vi "外观 2.vi"(0 "Data In":T6 caption="数据输入" format="%04x", 2 "Display State In":T4={"阀口名称"={"阀口名称自定义类型"=enum."自定义", "阀口自定义名称"={"V1"="V1", "V2"="V2", "V3"="V3", "V4"="V4", "V5"="V5", "V6"="V6", "V7"="V7", "V8"="V8", "V9"="V9", "V10"="V10", "V11"="V11", "V12"="V12", "V9-1"="V9-1", "V9-2"="V9-2", "COD慢速"="V9-2"}}} caption="显示状态输入", 3 "Container State":T5 caption="容器状态") -> (6 "Data Out":T6 caption="数据输出" format="%04x", 7 "Display State Out":T4={"阀口名称"={"阀口名称自定义类型"=enum."自定义", "阀口自定义名称"={"V1"="V1", "V2"="V2", "V3"="V3", "V4"="V4", "V5"="V5", "V6"="V6", "V7"="V7", "V8"="V8", "V9"="V9", "V10"="V10", "V11"="V11", "V12"="V12", "V9-1"="V9-1", "V9-2"="V9-2", "COD慢速"="V9-2"}}} caption="显示状态输出", 8 "Action":T3 caption="动作")   [LabVIEW 2016, in "调试控件V3.xctl"]
uses:
  <vilib>/_xctls/Container State.ctl
  <vilib>/_xctls/Action.ctl
  <vilib>/_xctls/XControlSupport.lvlib
panel:
  in  "项目输入":u16(ring) items=["总磷", "总氮", "氨氮", "磷酸盐", "硝氮", "亚硝氮", "硅酸盐", "硫化物", "COD"]
  in  "氨氮控温":bool
  in  "电磁阀2":bool
  in  "电磁阀1":bool
  in  "蠕动泵":bool
  in  "控温":enum32{"未选择", "消解", "恒温", "降温"}(radio)
  out "选项卡控件":enum32{"选项卡 1", "选项卡 2"}(tab)
  in  "COD慢速":bool
  in  "阀口选择":T1(radio)
  in  "V9-1":bool
  in  "V9-2":bool
  in  "灯":enum32{"未选择", "365", "520", "660", "氙灯/紫灯"}(radio)
  in  "ADC值":T2(radio)
  in  "注射泵":enum32{"等待", "复位", "注入", "注出"}(radio)=enum."注入"
  in  "数值":i16=4000
  # "外设"
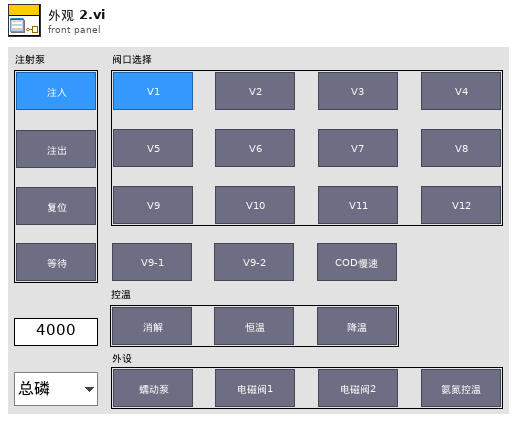
[diagram p1: front panel]
types:
  T1 = enum32{"V1", "V2", "V3", "V4", "V5", "V6", "V7", "V8", "V9", "V10", "V11", "V12"}
  T2 = enum32{"未选择", "ADC365", "ADC520", "ADC660", "光谱仪"}
  T3 = typedef "XControlSupport.lvlib/Action.ctl" = cluster{"Data Changed?":bool, "State Changed?":bool, "Action Name":string}
  T4 = typedef "调试控件V3.xctl/状态 2.ctl" = cluster{"阀口名称":cluster{"阀口名称自定义类型":enum16{"自定义", "微站总磷总氮", "微站总磷氨氮", "微站氨氮", "固定站总磷", "固定站总氮", "固定站氨氮", "原位总磷总氮", "原位总磷氨氮", "原位总磷", "原位总氮", "原位氨氮", "原位3N1P"}, "阀口自定义名称":cluster{"V1":string, "V2":string, "V3":string, "V4":string, "V5":string, "V6":string, "V7":string, "V8":string, "V9":string, "V10":string, "V11":string, "V12":string, "V9-1":string, "V9-2":string, "COD慢速":string}}}
  T5 = typedef "XControlSupport.lvlib/Container State.ctl" = cluster{"Indicator?":bool, "Run Mode?":bool, " Refnum":refnum<vi>}
  T6 = typedef "调试控件V3.xctl/数据 2.ctl" = u16[]
  T7 = cluster{"默认名称":cluster{"V1":string, "V2":string, "V3":string, "V4":string, "V5":string, "V6":string, "V7":string, "V8":string, "V9":string, "V10":string, "V11":string, "V12":string, "V9-1":string, "V9-2":string, "COD慢速":string}, "微站总磷总氮":cluster{"V1":string, "V2":string, "V3":string, "V4":string, "V5":string, "V6":string, "V7":string, "V8":string, "V9":string, "V10":string, "V11":string, "V12":string, "V9-1":string, "V9-2":string, "COD慢速":string}, "微站总磷氨氮":cluster{"V1":string, "V2":string, "V3":string, "V4":string, "V5":string, "V6":string, "V7":string, "V8":string, "V9":string, "V10":string, "V11":string, "V12":string, "V9-1":string, "V9-2":string, "COD慢速":string}, "微站氨氮":cluster{"V1":string, "V2":string, "V3":string, "V4":string, "V5":string, "V6":string, "V7":string, "V8":string, "V9":string, "V10":string, "V11":string, "V12":string, "V9-1":string, "V9-2":string, "COD慢速":string}, "固定站总磷":cluster{"V1":string, "V2":string, "V3":string, "V4":string, "V5":string, "V6":string, "V7":string, "V8":string, "V9":string, "V10":string, "V11":string, "V12":string, "V9-1":string, "V9-2":string, "COD慢速":string}, "固定站总氮":cluster{"V1":string, "V2":string, "V3":string, "V4":string, "V5":string, "V6":string, "V7":string, "V8":string, "V9":string, "V10":string, "V11":string, "V12":string, "V9-1":string, "V9-2":string, "COD慢速":string}, "固定站氨氮":cluster{"V1":string, "V2":string, "V3":string, "V4":string, "V5":string, "V6":string, "V7":string, "V8":string, "V9":string, "V10":string, "V11":string, "V12":string, "V9-1":string, "V9-2":string, "COD慢速":string}, "原位总磷总氮":cluster{"V1":string, "V2":string, "V3":string, "V4":string, "V5":string, "V6":string, "V7":string, "V8":string, "V9":string, "V10":string, "V11":string, "V12":string, "V9-1":string, "V9-2":string, "COD慢速":string}, "原位总磷氨氮":cluster{"V1":string, "V2":string, "V3":string, "V4":string, "V5":string, "V6":string, "V7":string, "V8":string, "V9":string, "V10":string, "V11":string, "V12":string, "V9-1":string, "V9-2":string, "COD慢速":string}, "原位总磷":cluster{"V1":string, "V2":string, "V3":string, "V4":string, "V5":string, "V6":string, "V7":string, "V8":string, "V9":string, "V10":string, "V11":string, "V12":string, "V9-1":string, "V9-2":string, "COD慢速":string}, "原位总氮":cluster{"V1":string, "V2":string, "V3":string, "V4":string, "V5":string, "V6":string, "V7":string, "V8":string, "V9":string, "V10":string, "V11":string, "V12":string, "V9-1":string, "V9-2":string, "COD慢速":string}, "原位氨氮":cluster{"V1":string, "V2":string, "V3":string, "V4":string, "V5":string, "V6":string, "V7":string, "V8":string, "V9":string, "V10":string, "V11":string, "V12":string, "V9-1":string, "V9-2":string, "COD慢速":string}, "原位3N1P":cluster{"V1":string, "V2":string, "V3":string, "V4":string, "V5":string, "V6":string, "V7":string, "V8":string, "V9":string, "V10":string, "V11":string, "V12":string, "V9-1":string, "V9-2":string, "COD慢速":string}}
  T8 = enum16{"自定义", "微站总磷总氮", "微站总磷氨氮", "微站氨氮", "固定站总磷", "固定站总氮", "固定站氨氮", "原位总磷总氮", "原位总磷氨氮", "原位总磷", "原位总氮", "原位氨氮", "原位3N1P"}
  T9 = cluster{"V1":string, "V2":string, "V3":string, "V4":string, "V5":string, "V6":string, "V7":string, "V8":string, "V9":string, "V10":string, "V11":string, "V12":string, "V9-1":string, "V9-2":string, "COD慢速":string}
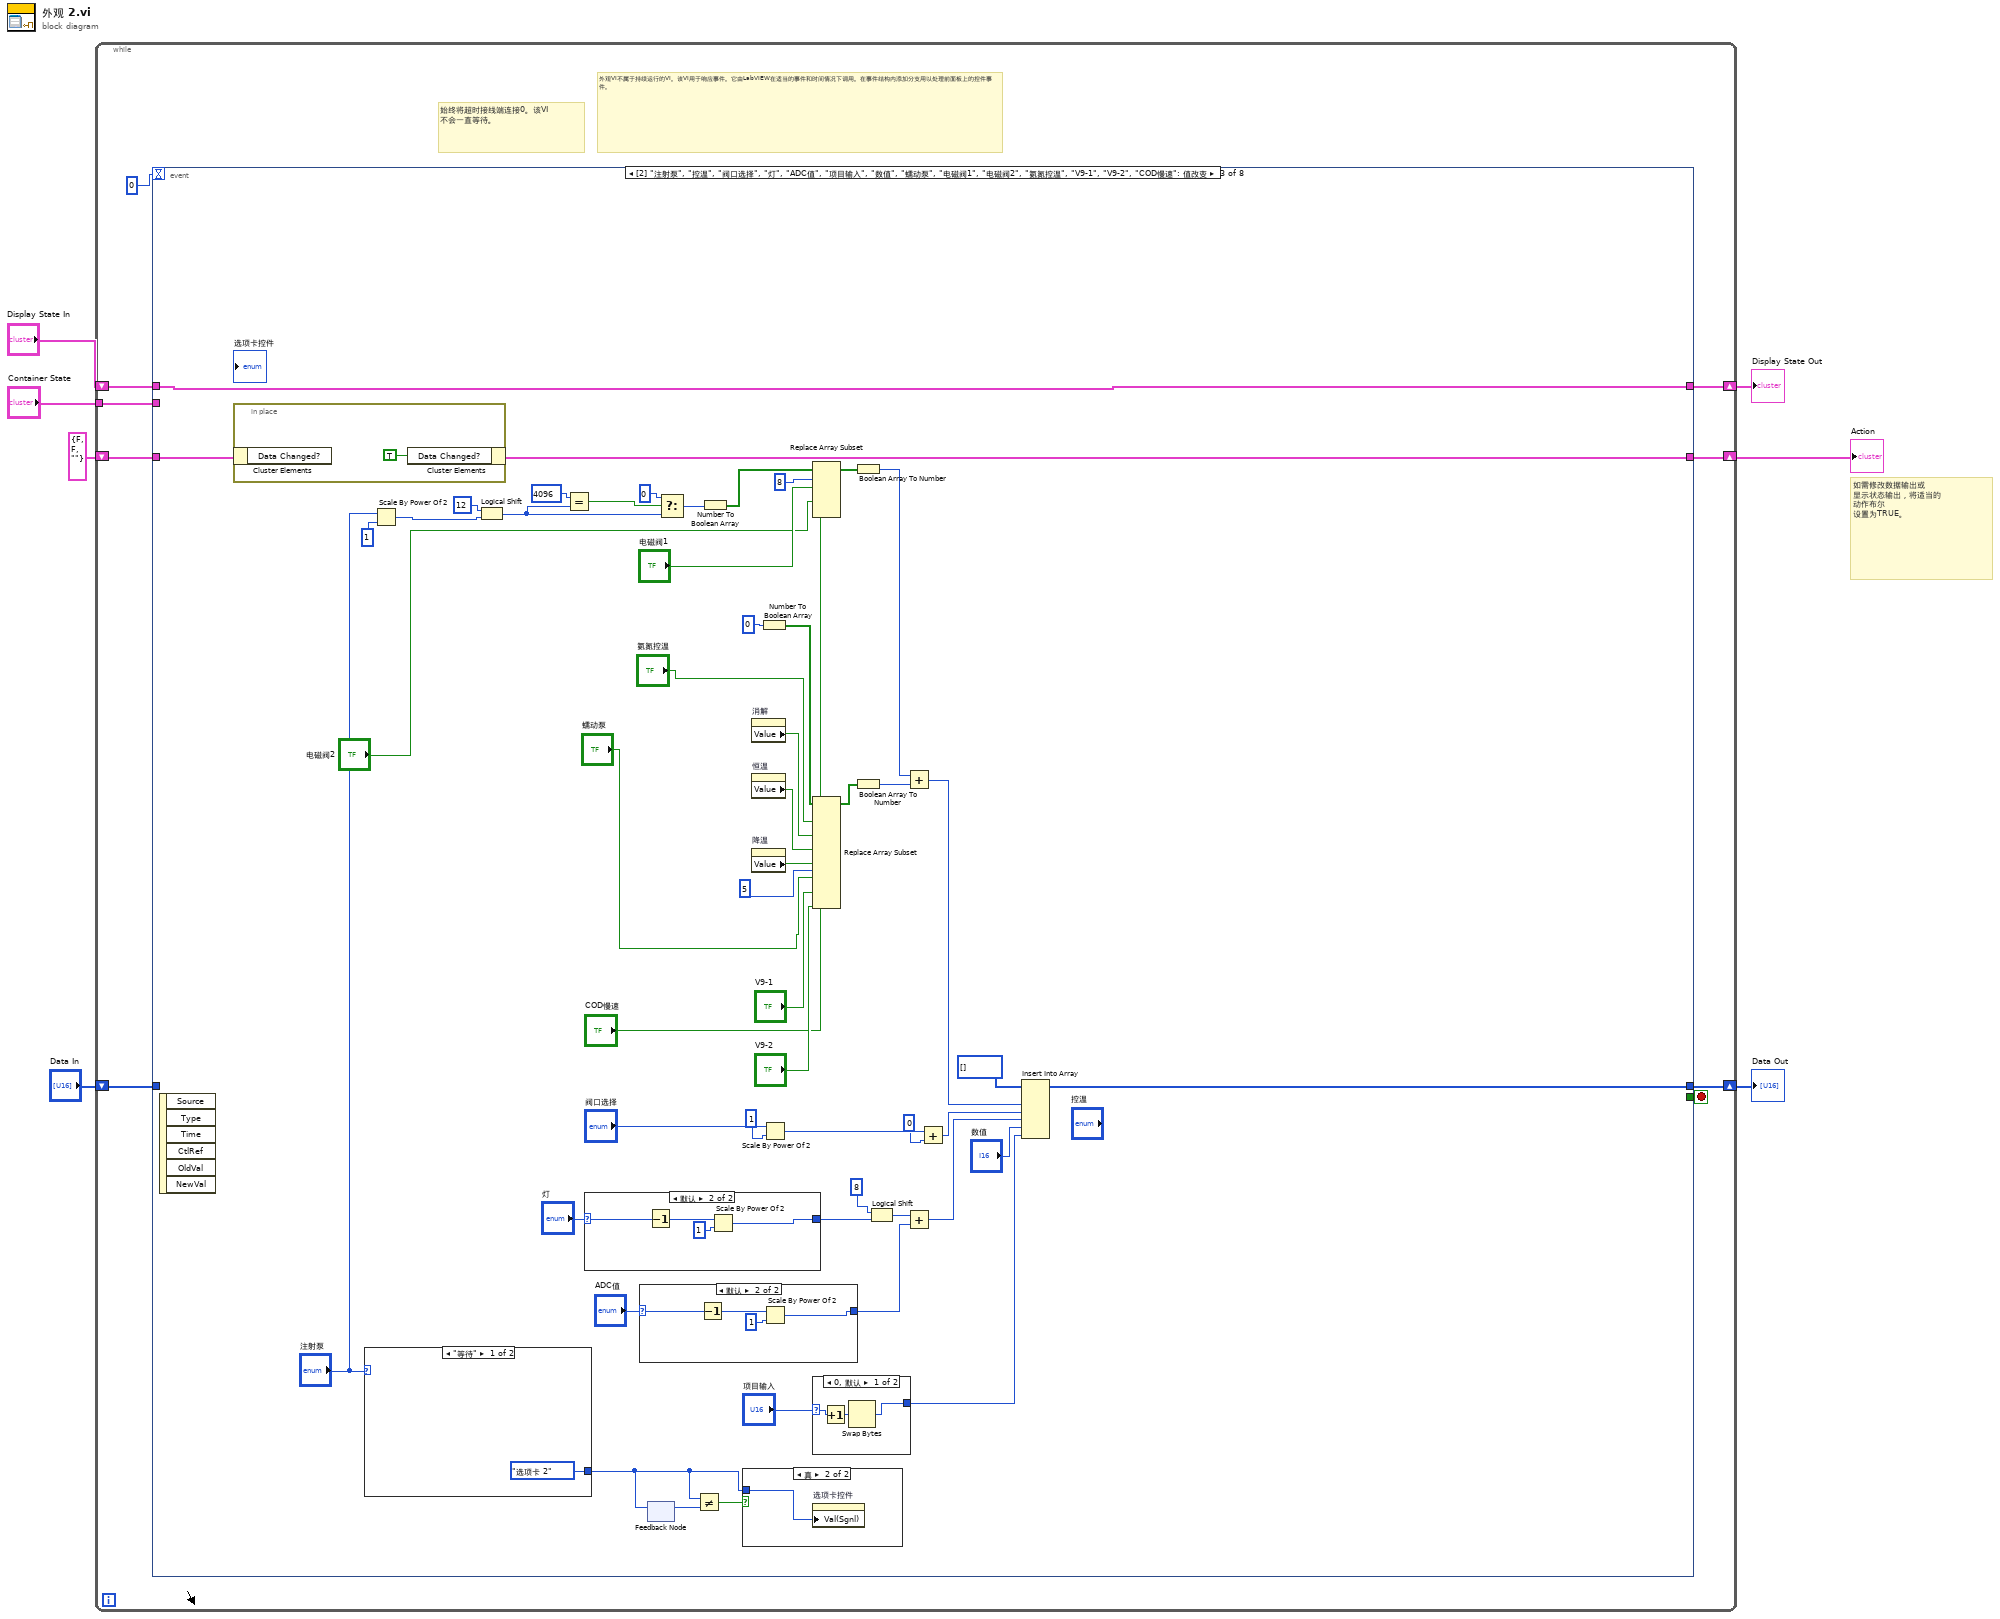
[diagram p0: block diagram]
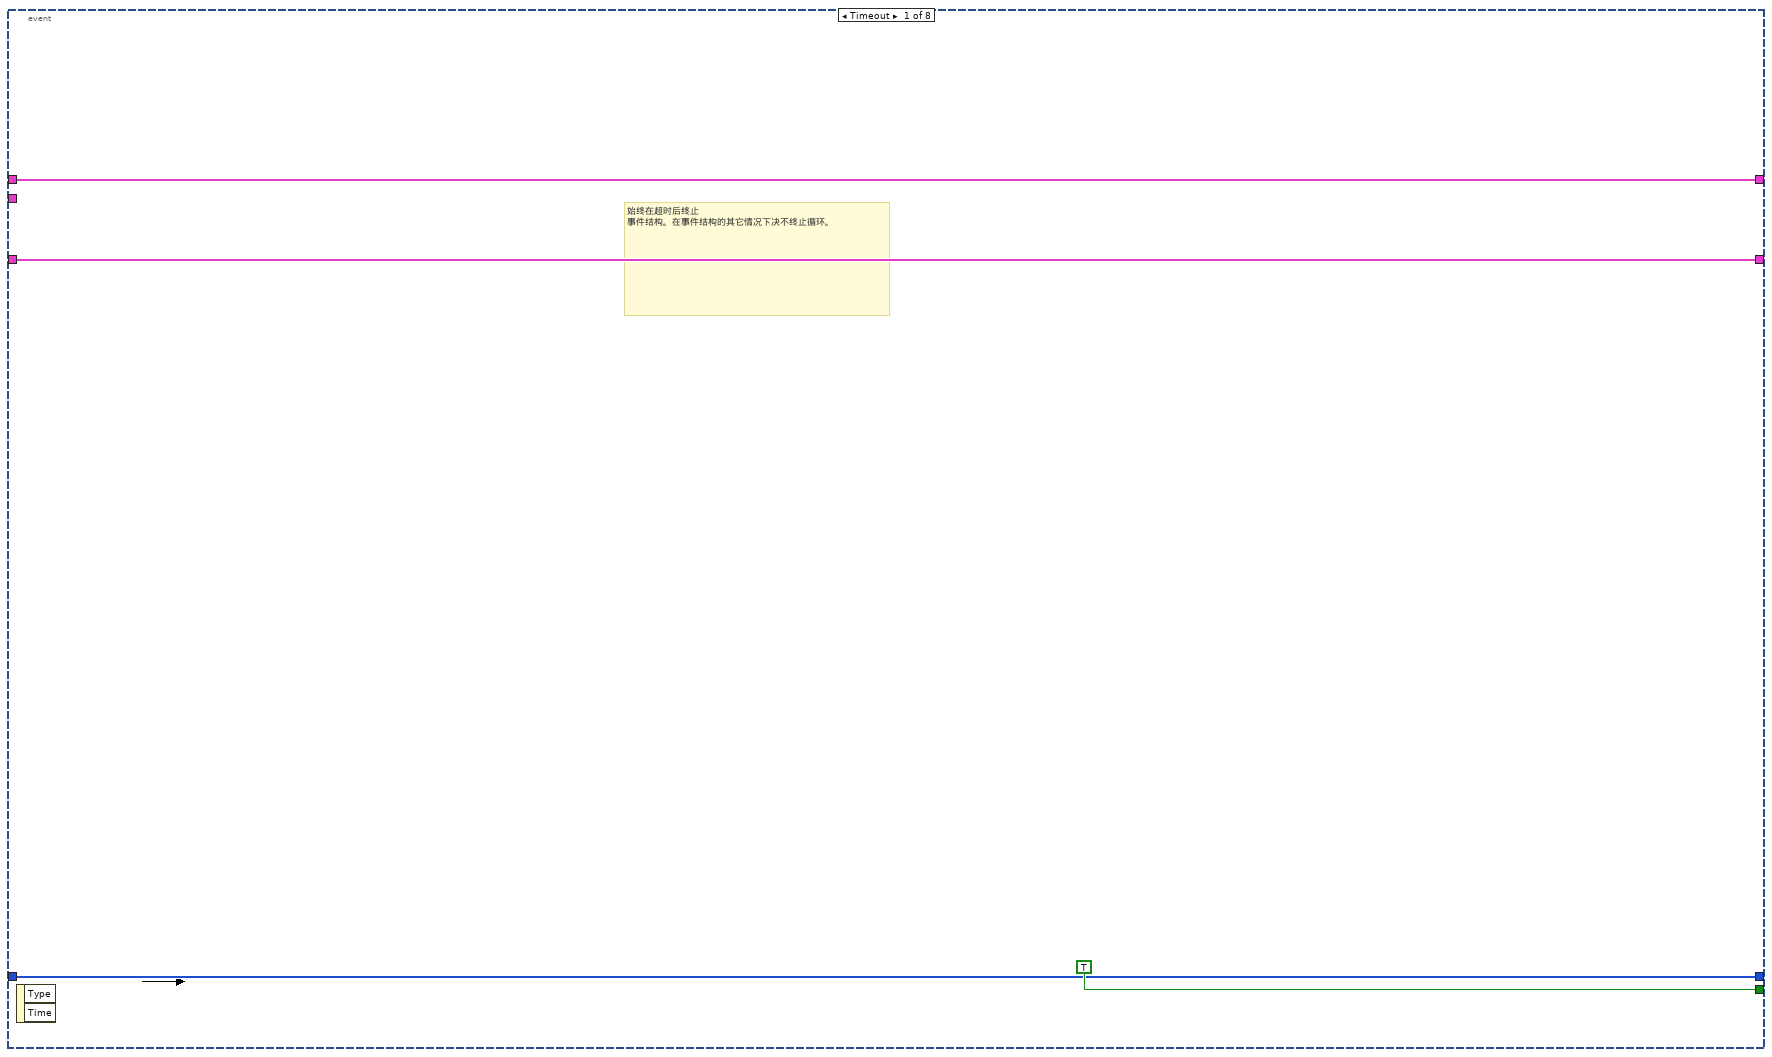
[diagram p2: hidden frame]
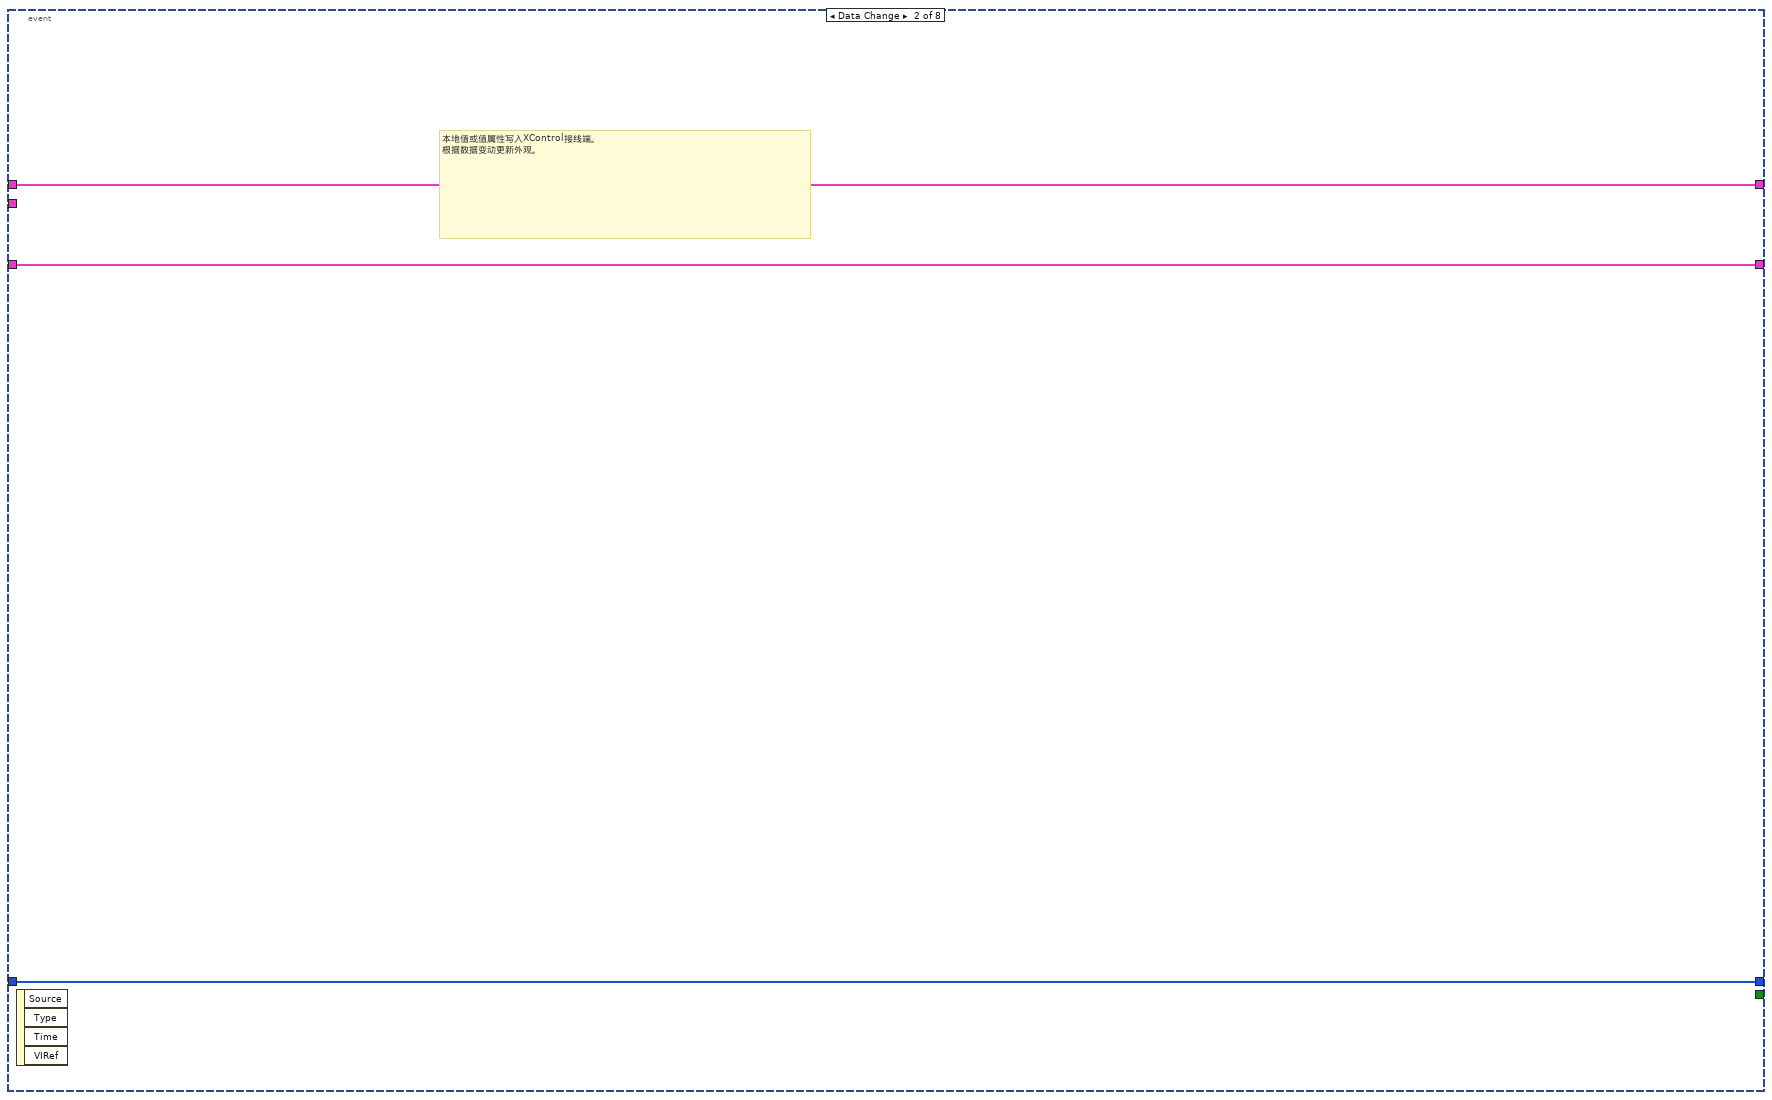
[diagram p3: hidden frame]
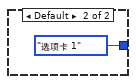
[diagram p5: hidden frame]
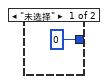
[diagram p6: hidden frame]
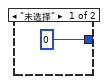
[diagram p7: hidden frame]
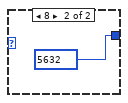
[diagram p8: hidden frame]
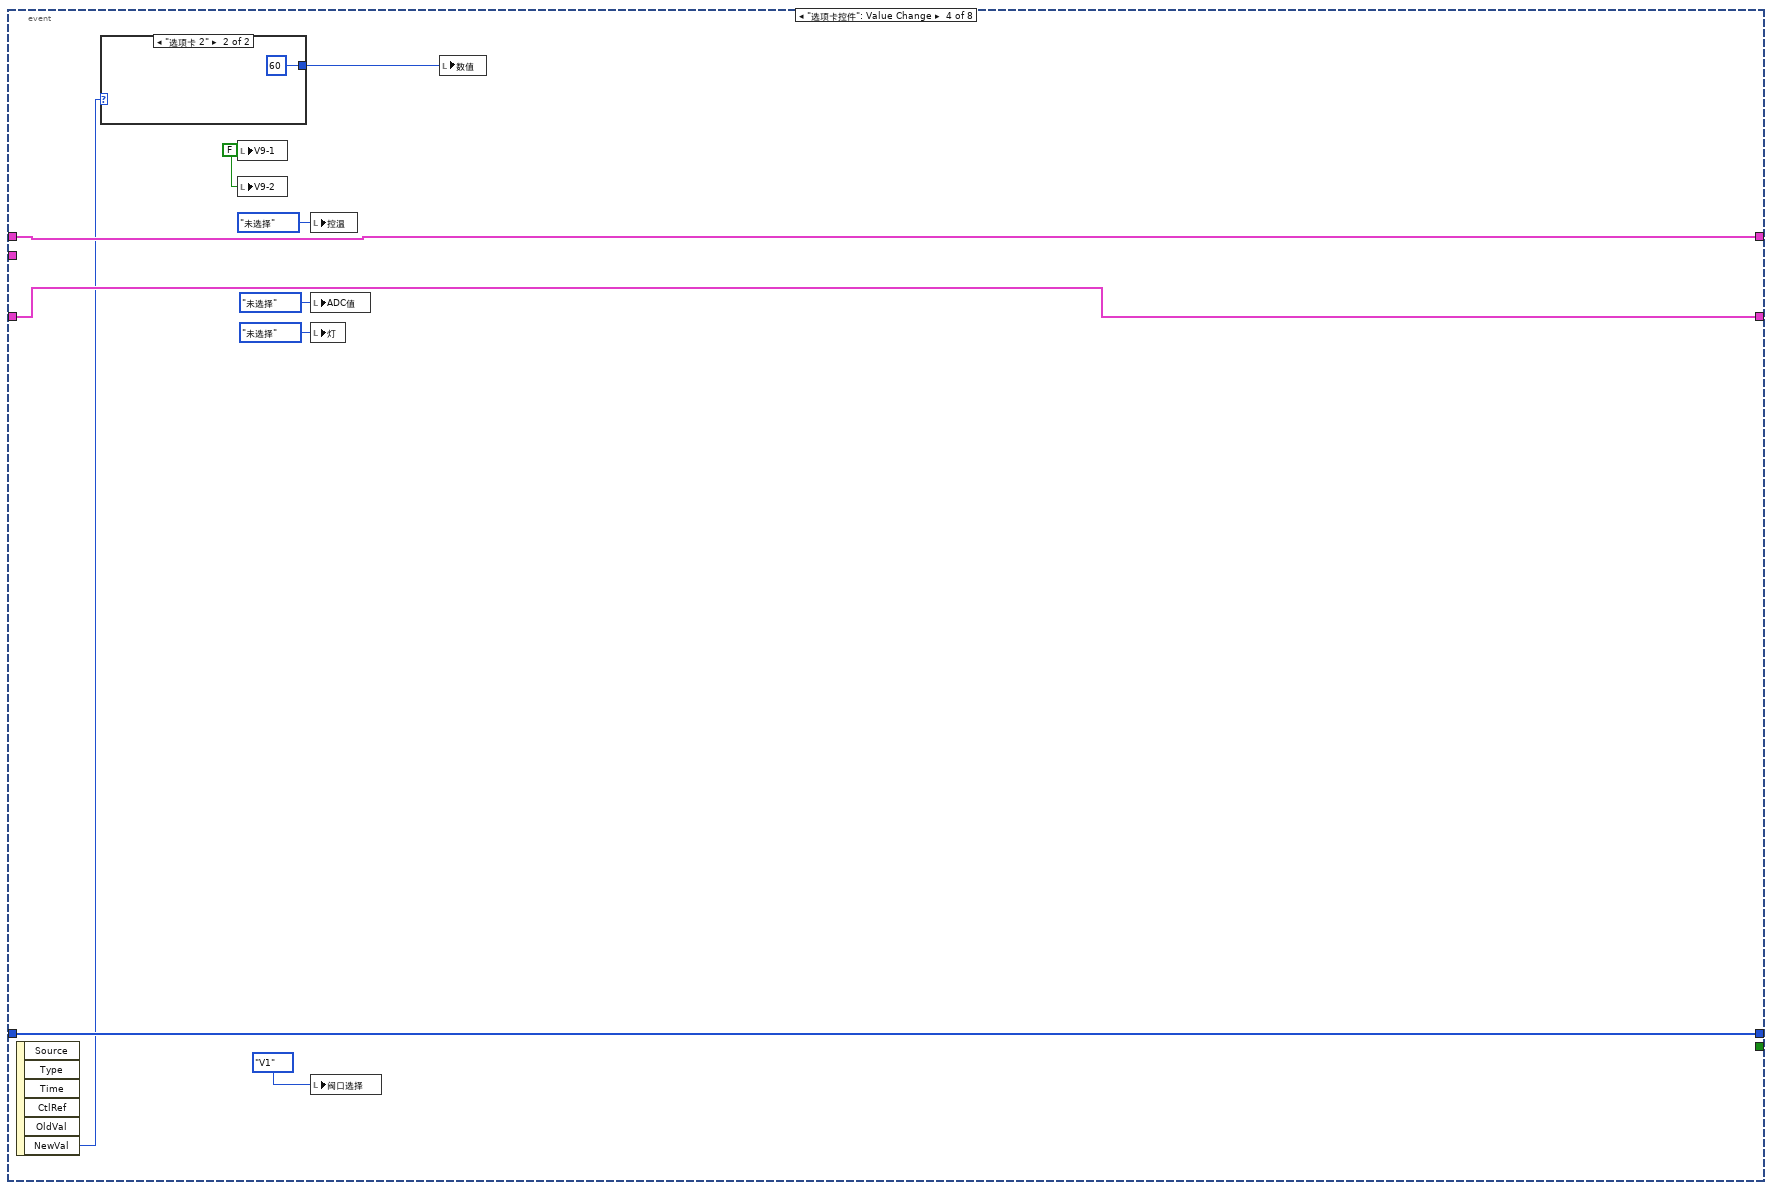
[diagram p9: hidden frame]
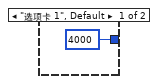
[diagram p10: hidden frame]
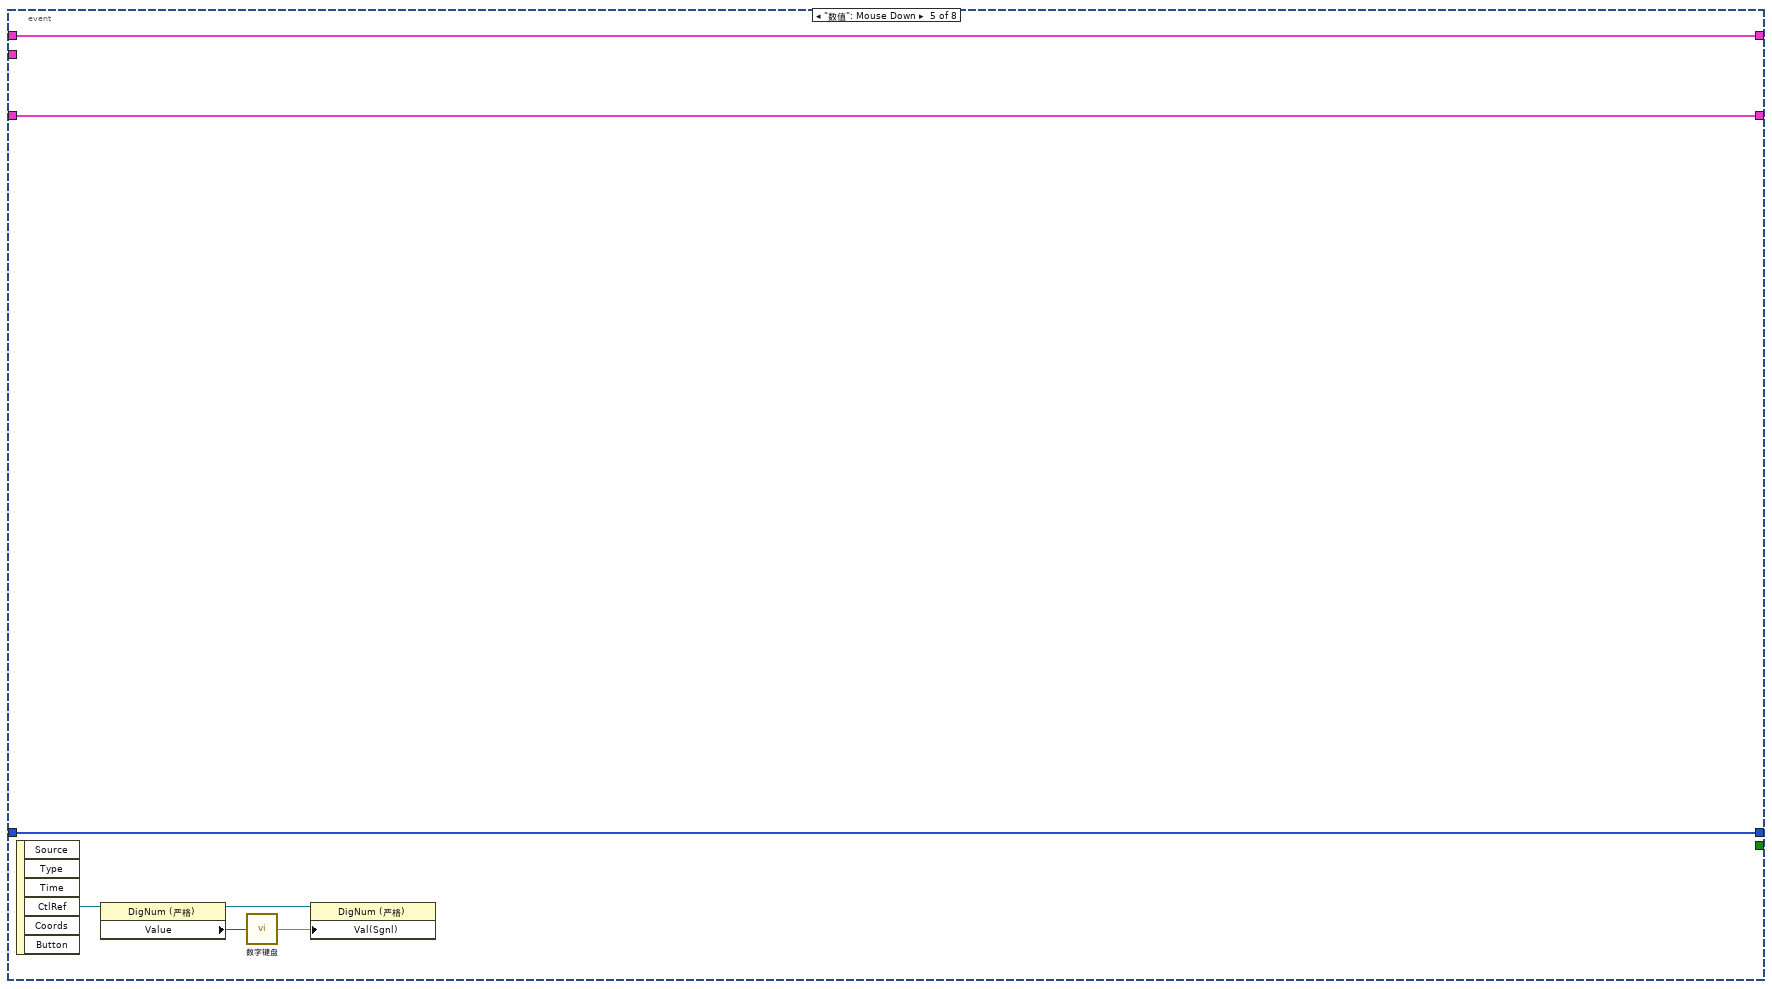
[diagram p11: hidden frame]
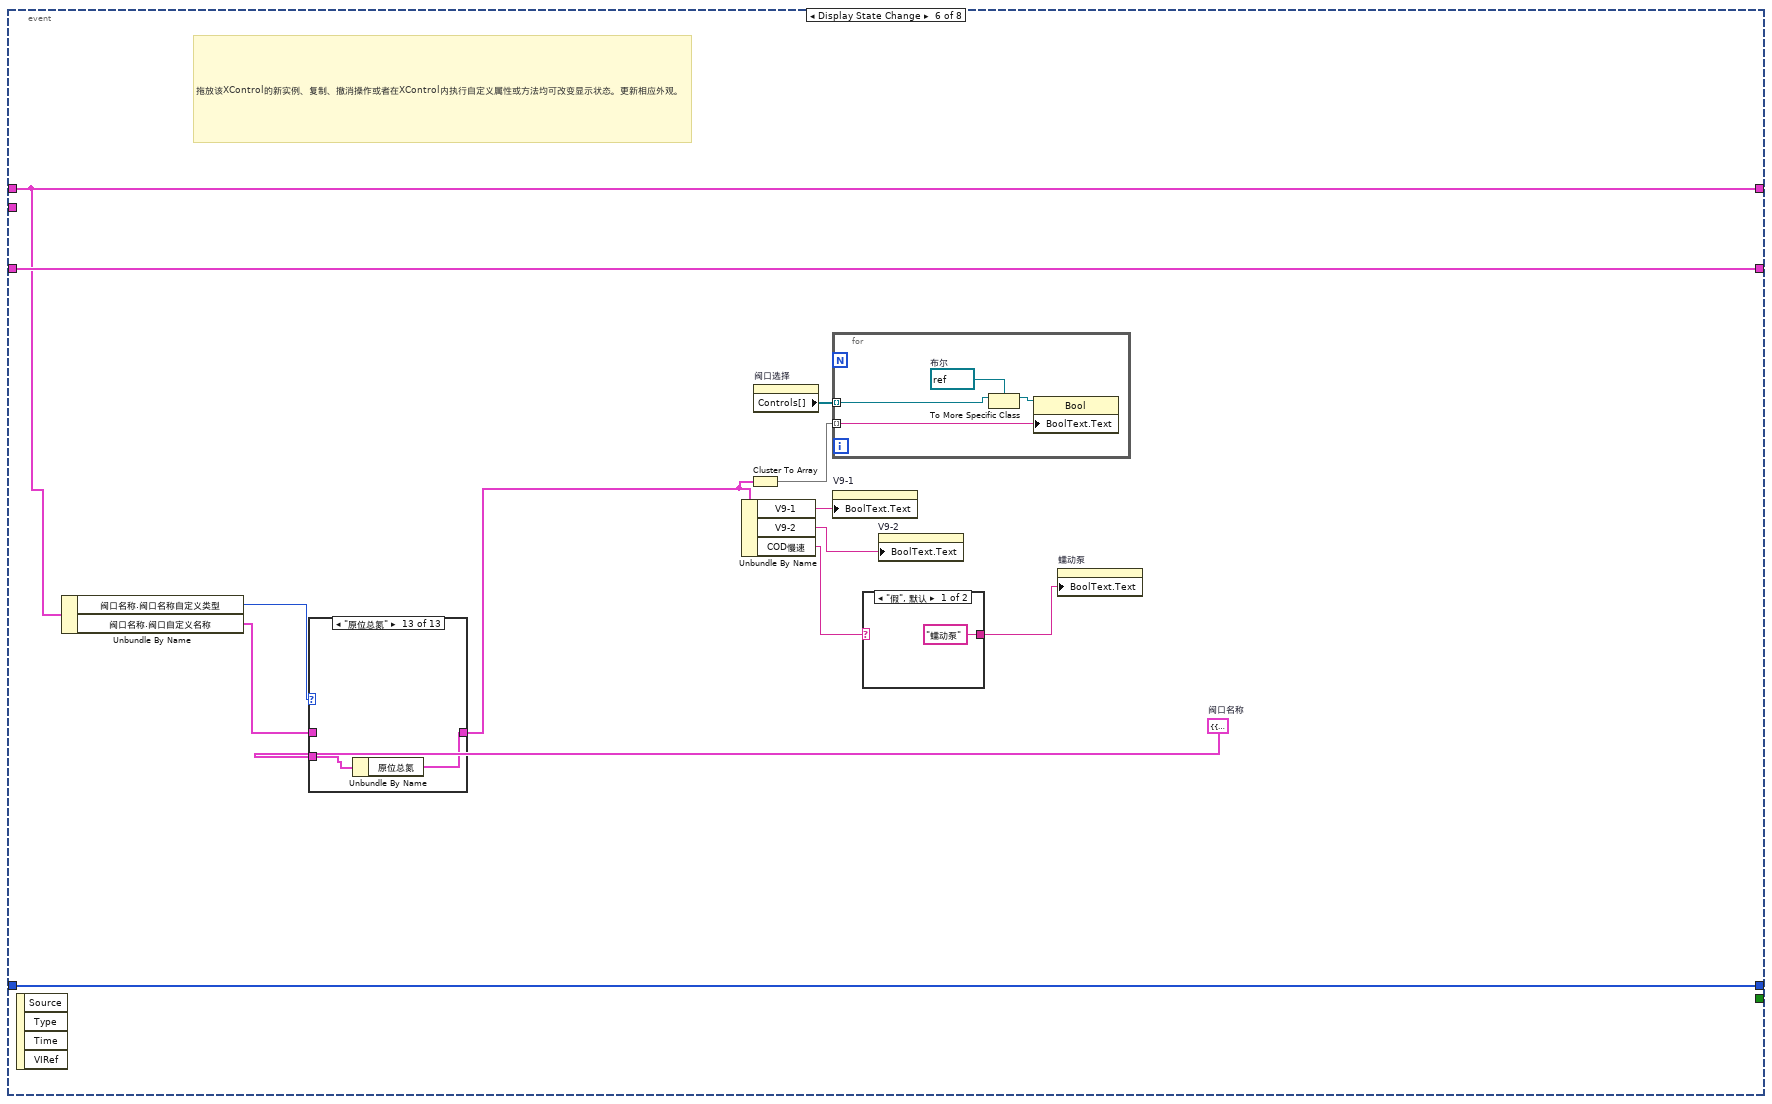
[diagram p12: hidden frame]
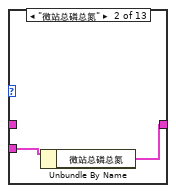
[diagram p15: hidden frame]
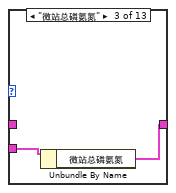
[diagram p16: hidden frame]
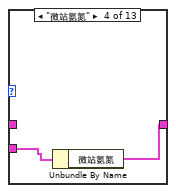
[diagram p17: hidden frame]
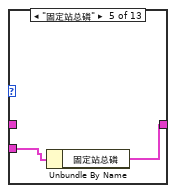
[diagram p18: hidden frame]
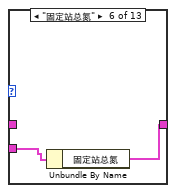
[diagram p19: hidden frame]
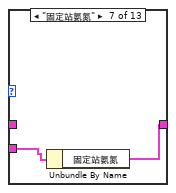
[diagram p20: hidden frame]
diagram:
  # "如需修改数据输出或\n显示状态输出，将适当的\n动作布尔\n设置为TRUE。"
  n1 = while {
    shift-right: [w15] -> w4
    shift-left: "Display State In" -> [w16]
    tunnel: "Container State" -> [w12]
    shift-right: [w10] -> w7
    shift-left: "Data In" -> [w11]
    shift-right: [w8] -> w2
    shift-left: T3 {"Data Changed?"=FALSE, "State Changed?"=FALSE, "Action Name"=""} ("Action") -> [w9]
    stop <- w14 stop-if-true
    # "外观VI不属于持续运行的VI。该VI用于响应事件。它由LabVIEW在适当的事件和时间情况下调用。在事件结构内添加分支用以处理前面板上的控件事件。"
    # "始终将超时接线端连接0。该VI\n不会一直等待。"
    n2 = event shown="[2] \"注射泵\", \"控温\", \"阀口选择\", \"灯\", \"ADC值\", \"项目输入\", \"数值\", \"蠕动泵\", \"电磁阀1\", \"电磁阀2\", \"氨氮控温\", \"V9-1\", \"V9-2\", \"COD慢速\": 值改变" {
      selector: _ -> [_ _ _ _ _ _ _ _]
      dyn-events: _ -> [_ _ _ _ _ _ _ _]
      timeout: 0 -> [_ _ _ _ _ _ _ _]
      tunnel: w16 -> [w18 w22 w75 w103 w112 w119 w159 w163]
      tunnel: [w18 w22 w75 w103 w112 w119 w159 w163] -> w15
      tunnel: [TRUE _ _ _ _ _ _ _] -> w14
      tunnel: w12 -> [_ _ _ _ _ _ w160 w164]
      tunnel: w11 -> [w17 w23 _ w102 w111 w125 w158 w162]
      tunnel: [w17 w23 w51 w102 w111 w125 w158 w162] -> w10
      tunnel: [w19 w21 w73 w101 w110 w124 w157 w161] -> w8
      tunnel: w9 -> [w19 w21 w74 w101 w110 w124 w157 w161]
      event Timeout {
        # "始终在超时后终止\n事件结构。在事件结构的其它情况下决不终止循环。"
        n3 = event-data() -> ()  [unwired: 1 in, 2 out]
      }
      event Data Change {
        # "本地值或值属性写入XControl接线端。\n根据数据变动更新外观。"
        n4 = event-data() -> ()  [unwired: 1 in, 4 out]
      }
      event "注射泵", "控温", "阀口选择", "灯", "ADC值", "项目输入", "数值", "蠕动泵", "电磁阀1", "电磁阀2", "氨氮控温", "V9-1", "V9-2", "COD慢速": Value Change {
        n5 = event-data() -> ()  [unwired: 1 in, 6 out]
        n6 = in-place {
          n7 = in-place-cluster #1(w74) -> ()  [unwired: 1 out]
          n8 = in-place-cluster #1("Data Changed?"=TRUE) -> (w73:T3)
        }
        n9 = case shown="\"等待\"" "注射泵" {
          tunnel: [enum32{"选项卡 1", "选项卡 2"}."选项卡 2" ("选项卡控件") enum32{"选项卡 1", "选项卡 2"}."选项卡 1" ("选项卡控件")] -> w45
          frame "等待" {
          }
          frame Default {
          }
        }
        n10 = Scale By Power Of 2(n="注射泵", x=i16 1 ("y")) -> (x*2^n=w59:i16)
        n11 = Logical Shift(y=i16 12, x=w59) -> (x << y=w64:i16)
        n12 = Equal?(x=u32 4096 ("t"), y=w64) -> (x = y?=w72:bool)
        n13 = case shown="默认" "灯" {
          selector: "灯" -> [_ w86]
          tunnel: [i16 0 ("y") w88] -> w56
          frame "未选择" {
          }
          frame Default {
            n14 = Decrement(x=w86) -> (x-1=w87:enum32{"未选择", "365", "520", "660", "氙灯/紫灯"})
            n15 = Scale By Power Of 2(n=w87, x=i16 1 ("y")) -> (x*2^n=w88:i16)
          }
        }
        n16 = case shown="默认" "ADC值" {
          selector: "ADC值" -> [_ w81]
          tunnel: [i16 0 ("y") w83] -> w55
          frame "未选择" {
          }
          frame Default {
            n17 = Decrement(x=w81) -> (x-1=w82:T2)
            n18 = Scale By Power Of 2(n=w82, x=i16 1 ("y")) -> (x*2^n=w83:i16)
          }
        }
        n19 = feedback-in #2(w45) -> ()
        n20 = feedback #2() -> (w47:enum32{"选项卡 1", "选项卡 2"})  [unwired: 1 in]
        n21 = Select(t=u32 0, s=w72, f=w64) -> (s? t:f=w41:u32)
        n22 = Not Equal?(x=w45, y=w47) -> (x != y?=w46:bool)
        n23 = Number To Boolean Array(number=w41) -> (Boolean array=w40:bool[])
        n24 = case shown="真" w46 {
          tunnel: w45 -> [_ w76]
          frame False {
          }
          frame True {
            n25 = property on="选项卡控件" class="TabCtl (严格)"("Val(Sgnl)"=w76) -> ()  [unwired: 2 in, 2 out]
          }
        }
        n26 = property on="消解" class="Bool (严格)"() -> ("Value"=w36:bool)  [unwired: 2 in, 2 out]
        n27 = property on="恒温" class="Bool (严格)"() -> ("Value"=w35:bool)  [unwired: 2 in, 2 out]
        n28 = property on="降温" class="Bool (严格)"() -> ("Value"=w34:bool)  [unwired: 2 in, 2 out]
        n29 = Number To Boolean Array(number=u16 0) -> (Boolean array=w31:bool[])
        n30 = Scale By Power Of 2(n="阀口选择", x=i16 1 ("y")) -> (x*2^n=w58:i16)
        n31 = Replace Array Subset(array=w40, new element #1="电磁阀1", index #1=8 ("索引"), new element #2="电磁阀2", new element #3="COD慢速") -> (w39:bool[])  [unwired: 2 in]
        n32 = Replace Array Subset(array=w31, new element #1="氨氮控温", new element #2=w36, new element #3=w35, new element #4=w34, new element #5="蠕动泵", index #5=5 ("索引"), new element #6="V9-1", new element #7="V9-2") -> (w48:bool[])  [unwired: 6 in]
        n33 = case shown="0, 默认" "项目输入" {
          selector: "项目输入" -> [w91 _]
          tunnel: [w90 5632] -> w61
          frame 0, Default {
            n34 = Increment(x=w91) -> (x+1=w89:u16)
            n35 = Swap Bytes(anything=w89) -> (byte swapped=w90:u16)
          }
          frame 8 {
          }
        }
        n36 = Boolean Array To Number(Boolean array=w39) -> (number=w38:u32)
        n37 = Boolean Array To Number(Boolean array=w48) -> (number=w44:u32)
        n38 = Logical Shift(y=i16 8, x=w56) -> (x << y=w70:i16)
        n39 = Add(x=w38, y=w44) -> (x+y=w67:u32)
        n40 = Add(x=w70, y=w55) -> (x+y=w66:i16)
        n41 = Add(x=w58, y=i16 0) -> (x+y=w57:i16)
        n42 = Insert Into Array(array=u16[] [] ("数组"), new element #1=w67, new element #2=w57, new element #3=w66, new element #4="数值", new element #5=w61) -> (w51:u16[])  [unwired: 1 in]
      }
      event "选项卡控件": Value Change {
        w97 = FALSE ("V9-1")
        n43 = event-data() -> ("NewVal"=w100:enum32{"选项卡 1", "选项卡 2"})  [unwired: 1 in, 5 out]
        n44 = case shown="\"选项卡 2\"" w100 {
          tunnel: [i16 4000 ("数值") i16 60 ("数值")] -> w99
          frame "选项卡 1", Default {
          }
          frame "选项卡 2" {
          }
        }
        n45 = local write "V9-1"(w97) -> ()
        n46 = local write "V9-2"(w97) -> ()
        n47 = local write "控温"(enum32{"未选择", "消解", "恒温", "降温"}."未选择" ("控温")) -> ()
        n48 = local write "ADC值"(T2."未选择" ("ADC值")) -> ()
        n49 = local write "灯"(enum32{"未选择", "365", "520", "660", "氙灯/紫灯"}."未选择" ("灯")) -> ()
        n50 = local write "阀口选择"(T1."V1" ("阀口选择")) -> ()
        n51 = local write "数值"(w99) -> ()
      }
      event "数值": Mouse Down {
        n52 = event-data() -> ("CtlRef"=w109:refnum<vi>)  [unwired: 1 in, 5 out]
        n53 = property class="DigNum (严格)"(reference=w109) -> (reference out=w108:refnum<vi>, "Value"=w107:i16)  [unwired: 1 in, 1 out]
        n54 = call "数字键盘.vi"("OldNumber"=w107) -> ("NewNumber"=w106:sgl)
        n55 = property class="DigNum (严格)"(reference=w108, "Val(Sgnl)"=w106) -> ()  [unwired: 1 in, 2 out]
      }
      event Display State Change {
        w116 = T7 {"默认名称"={"V1"="V1", "V2"="V2", "V3"="V3", "V4"="V4", "V5"="V5", "V6"="V6", "V7"="V7", "V8"="V8", "V9"="V9", "V10"="V10", "V11"="V11", "V12"="V12", "V9-1"="V9-1", "V9-2"="V9-2", "COD慢速"="COD慢速"}, "微站总磷总氮"={"V1"="TA", "V2"="TB", "V3"="TC", "V4"="PA", "V5"="PB", "V6"="零点核查", "V7"="跨度核查", "V8"="纯水", "V9"="水样", "V10"="消解", "V11"="总氮比色", "V12"="总磷比色/废液", "V9-1"="加标回收", "V9-2"="标样核查", "COD慢速"="COD慢速"}, "微站总磷氨氮"={"V1"="NA", "V2"="NB", "V3"="NC", "V4"="TB", "V5"="PA", "V6"="PB", "V7"="跨度核查", "V8"="纯水", "V9"="水样", "V10"="消解", "V11"="空气", "V12"="比色/废液", "V9-1"="加标回收", "V9-2"="标样核查", "COD慢速"="COD慢速"}, "微站氨氮"={"V1"="NA", "V2"="NB", "V3"="NC", "V4"="零点核查", "V5"="跨度核查", "V6"="空气", "V7"="纯水", "V8"="水样", "V9"="排液", "V10"="V10", "V11"="V11", "V12"="V12", "V9-1"="加标回收", "V9-2"="标样核查", "COD慢速"="COD慢速"}, "固定站总磷"={"V1"="TB", "V2"="PA", "V3"="PB", "V4"="排液", "V5"="标样核查", "V6"="零点核查", "V7"="跨度核查", "V8"="纯水", "V9"="水样/加标", "V10"="消解", "V11"="空气", "V12"="总磷比色/废液", "V9-1"="V9-1", "V9-2"="V9-2", "COD慢速"="COD慢速"}, "固定站总氮"={"V1"="TA", "V2"="TB", "V3"="TC", "V4"="排液", "V5"="标样核查", "V6"="零点核查", "V7"="跨度核查", "V8"="纯水", "V9"="水样/加标", "V10"="消解", "V11"="总氮比色", "V12"="废液", "V9-1"="V9-1", "V9-2"="V9-2", "COD慢速"="COD慢速"}, "固定站氨氮"={"V1"="NA", "V2"="NB", "V3"="NC", "V4"="零点核查", "V5"="跨度核查", "V6"="空气", "V7"="纯水", "V8"="水样", "V9"="排液", "V10"="V10", "V11"="V11", "V12"="V12", "V9-1"="加标回收", "V9-2"="标样核查", "COD慢速"="COD慢速"}, "原位总磷总氮"={"V1"="TA", "V2"="TB", "V3"="TC", "V4"="PA", "V5"="PB", "V6"="零点核查", "V7"="跨度核查", "V8"="纯水", "V9"="水样", "V10"="消解", "V11"="总氮比色", "V12"="总磷比色/废液", "V9-1"="V9-1", "V9-2"="V9-2", "COD慢速"="COD慢速"}, "原位总磷氨氮"={"V1"="NA", "V2"="NB", "V3"="NC", "V4"="TB", "V5"="PA", "V6"="PB", "V7"="跨度核查", "V8"="纯水", "V9"="水样", "V10"="消解", "V11"="空气", "V12"="比色/废液", "V9-1"="V9-1", "V9-2"="V9-2", "COD慢速"="COD慢速"}, "原位总磷"={"V1"="TB", "V2"="PA", "V3"="PB", "V4"="排液", "V5"="标样核查", "V6"="零点核查", "V7"="跨度核查", "V8"="纯水", "V9"="水样/加标", "V10"="消解", "V11"="空气", "V12"="总磷比色/废液", "V9-1"="V9-1", "V9-2"="V9-2", "COD慢速"="COD慢速"}, "原位总氮"={"V1"="TA", "V2"="TB", "V3"="TC", "V4"="排液", "V5"="标样核查", "V6"="零点核查", "V7"="跨度核查", "V8"="纯水", "V9"="水样/加标", "V10"="消解", "V11"="总氮比色", "V12"="废液", "V9-1"="V9-1", "V9-2"="V9-2", "COD慢速"="COD慢速"}, "原位氨氮"={"V1"="NA", "V2"="NB", "V3"="NC", "V4"="零点核查", "V5"="跨度核查", "V6"="空气", "V7"="纯水", "V8"="水样", "V9"="排液", "V10"="V10", "V11"="V11", "V12"="V12", "V9-1"="加标回收", "V9-2"="标样核查", "COD慢速"="COD慢速"}, "原位3N1P"={"V1"="NAB", "V2"="PA", "V3"="PB", "V4"="OA", "V5"="OB", "V6"="RA", "V7"="空气", "V8"="纯水", "V9"="水样", "V10"="紫外还原", "V11"="氨氮比色", "V12"="排液/比色", "V9-1"="V9-1", "V9-2"="V9-2", "COD慢速"="COD慢速"}}  # 阀口名称
        # "拖放该XControl的新实例、复制、撤消操作或者在XControl内执行自定义属性或方法均可改变显示状态。更新相应外观。"
        n56 = event-data() -> ()  [unwired: 1 in, 4 out]
        n57 = Unbundle By Name(w119) -> ("阀口名称.阀口名称自定义类型"=w118:T8, "阀口名称.阀口自定义名称"=w117:T9)
        n58 = case shown="\"原位总氮\"" w118 {
          tunnel: w117 -> [w128 _ _ _ _ _ _ _ _ _ _ _ _]
          tunnel: [w128 w129 w131 w133 w135 w137 w139 w141 w143 w145 w147 w149 w151] -> w115
          tunnel: w116 -> [_ w130 w132 w134 w136 w138 w140 w142 w144 w146 w148 w150 w152]
          frame "自定义", Default {
          }
          frame "微站总磷总氮" {
            n59 = Unbundle By Name(w130) -> ("微站总磷总氮"=w129:T9)
          }
          frame "微站总磷氨氮" {
            n60 = Unbundle By Name(w132) -> ("微站总磷氨氮"=w131:T9)
          }
          frame "微站氨氮" {
            n61 = Unbundle By Name(w134) -> ("微站氨氮"=w133:T9)
          }
          frame "固定站总磷" {
            n62 = Unbundle By Name(w136) -> ("固定站总磷"=w135:T9)
          }
          frame "固定站总氮" {
            n63 = Unbundle By Name(w138) -> ("固定站总氮"=w137:T9)
          }
          frame "固定站氨氮" {
            n64 = Unbundle By Name(w140) -> ("固定站氨氮"=w139:T9)
          }
          frame "原位总磷总氮" {
            n65 = Unbundle By Name(w142) -> ("原位总磷总氮"=w141:T9)
          }
          frame "原位总磷氨氮" {
            n66 = Unbundle By Name(w144) -> ("原位总磷氨氮"=w143:T9)
          }
          frame "原位总磷" {
            n67 = Unbundle By Name(w146) -> ("原位总磷"=w145:T9)
          }
          frame "原位氨氮" {
            n68 = Unbundle By Name(w148) -> ("原位氨氮"=w147:T9)
          }
          frame "原位3N1P" {
            n69 = Unbundle By Name(w150) -> ("原位3N1P"=w149:T9)
          }
          frame "原位总氮" {
            n70 = Unbundle By Name(w152) -> ("原位总氮"=w151:T9)
          }
        }
        n71 = Unbundle By Name(w115) -> ("V9-1"=w121:string, "V9-2"=w120:string, "COD慢速"=w114:string)
        n72 = Cluster To Array(cluster=w115) -> (array=w122:string[])
        n73 = property on="阀口选择" class="RadioBtnsControl (严格)"() -> ("Controls[]"=w123:refnum<vi>[])  [unwired: 2 in, 2 out]
        n74 = for {
          tunnel: w123 -> [w156] mode=indexing
          tunnel: w122 -> [w153] mode=indexing
          w155 = refnum<vi> refnum  # 布尔
          n75 = To More Specific Class(target class=w155, reference=w156) -> (specific class reference=w154:refnum<vi>)  [unwired: 1 in, 1 out]
          n76 = property class="Bool"(reference=w154, "BoolText.Text"=w153) -> ()  [unwired: 1 in, 2 out]
        }
        n77 = property on="V9-1" class="Bool (严格)"("BoolText.Text"=w121) -> ()  [unwired: 2 in, 2 out]
        n78 = case shown="\"假\", 默认" w114 {
          selector: w114 -> [_ w127]
          tunnel: ["蠕动泵" w127] -> w113
          frame "假", Default {
          }
          frame "风扇" {
          }
        }
        n79 = property on="V9-2" class="Bool (严格)"("BoolText.Text"=w120) -> ()  [unwired: 2 in, 2 out]
        n80 = property on="蠕动泵" class="Bool (严格)"("BoolText.Text"=w113) -> ()  [unwired: 2 in, 2 out]
      }
      event Direction Change {
        # "XControl的方向由输入控件转换为显示控件，反之亦然。更新相应外观。"
        n81 = event-data() -> ()  [unwired: 1 in, 4 out]
        n82 = Unbundle By Name(w160) -> ()  [unwired: 1 out]
      }
      event Exec State Change {
        # "包含该XControl的VI已从编辑模式切换至运行模式，反之亦然。\n相应的更新外观。"
        # "分别处理编辑模式和\n运行模式"
        n83 = event-data() -> ()  [unwired: 1 in, 4 out]
        n84 = Unbundle By Name(w164) -> ()  [unwired: 1 out]
      }
    }
  }
  "Display State Out" <- w4
  "Data Out" <- w7
  "Action" <- w2
